vi "parse_endpoint_state_roslv.vi"(4 "error in":errorcluster, 7 "msg in":string) -> (0 "error out":errorcluster, 2 "Endpoint State":T1, 3 "msg out":string)   [LabVIEW 2014]
doc: "Parses a message into endpoint states"
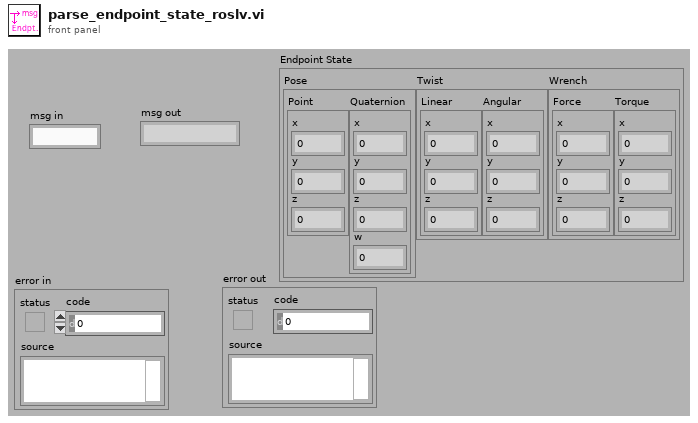
[diagram p1: front panel]
types:
  T1 = cluster{"Pose":cluster{"Point":cluster{"x":dbl, "y":dbl, "z":dbl}, "Quaternion":cluster{"x":dbl, "y":dbl, "z":dbl, "w":dbl}}, "Twist":cluster{"Linear":cluster{"x":dbl, "y":dbl, "z":dbl}, "Angular":cluster{"x":dbl, "y":dbl, "z":dbl}}, "Wrench":cluster{"Force":cluster{"x":dbl, "y":dbl, "z":dbl}, "Torque":cluster{"x":dbl, "y":dbl, "z":dbl}}}
  T2 = cluster{"Point":cluster{"x":dbl, "y":dbl, "z":dbl}, "Quaternion":cluster{"x":dbl, "y":dbl, "z":dbl, "w":dbl}}
  T3 = cluster{"Linear":cluster{"x":dbl, "y":dbl, "z":dbl}, "Angular":cluster{"x":dbl, "y":dbl, "z":dbl}}
  T4 = cluster{"Force":cluster{"x":dbl, "y":dbl, "z":dbl}, "Torque":cluster{"x":dbl, "y":dbl, "z":dbl}}
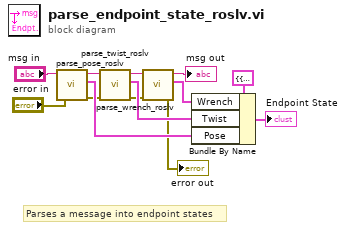
[diagram p0: block diagram]
diagram:
  # "Parses a message into endpoint states"
  n1 = call "parse_pose_roslv.vi"("error in"="error in", "msg in"="msg in") -> ("error out"=w4:errorcluster, "Pose"=w8:T2, "msg out"=w13:string)  [unwired: 3 in]
  n2 = call "parse_twist_roslv.vi"("error in"=w4, "msg in"=w13) -> ("error out"=w3:errorcluster, "Twist"=w9:T3, "msg out"=w12:string)  [unwired: 3 in]
  n3 = call "parse_wrench_roslv.vi"("error in"=w3, "msg in"=w12) -> ("error out"=→"error out":errorcluster, "Wrench"=w10:T4, "msg out"=→"msg out":string)  [unwired: 3 in]
  n4 = Bundle By Name(cluster=T1 {"Pose"={"Point"={"x"=0.0, "y"=0.0, "z"=0.0}, "Quaternion"={"x"=0.0, "y"=0.0, "z"=0.0, "w"=0.0}}, "Twist"={"Linear"={"x"=0.0, "y"=0.0, "z"=0.0}, "Angular"={"x"=0.0, "y"=0.0, "z"=0.0}}, "Wrench"={"Force"={"x"=0.0, "y"=0.0, "z"=0.0}, "Torque"={"x"=0.0, "y"=0.0, "z"=0.0}}} ("Endpoint State"), "Wrench"=w10, "Twist"=w9, "Pose"=w8) -> (→"Endpoint State":T1)
